vi "JSON Test.vi"() -> ()   [LabVIEW 2017]
uses:
  Classes/JSON Builder/JSON Builder.lvclass
  Typedefs/DSF Engine Framework Configuration.ctl
  DSF Core.lvlib
  Typedefs/DSF Engine Plugin Configuration.ctl
  Typedefs/DSF Timing Info.ctl
  Typedefs/DSF Engine Plugin Thread Configuration.ctl
  Typedefs/DSF Settings Info.ctl
  Typedefs/DSF Engine Transfer Group Configuration.ctl
  Typedefs/DSF Direction.ctl
  Typedefs/DSF Engine Transfer Configuration.ctl
  Typedefs/DSF Byte Order.ctl
  Typedefs/DSF Engine Channel Configuration.ctl
  Typedefs/DSF Data Type.ctl
  Typedefs/DSF Timeout Behavior.ctl
panel:
  out "Framework Configuration out":T1
  in  "Framework Configuration in":T1={"Plugins"=[{"name"="UDP", "components"=["UDP"], "cycle timing"={"priority"=100, "decimation"=1, "offset"=0}, "threads"=[{"buffer converter settings"=[], "transceiver settings"=[{"key"="Local Port", "value"="50000"}], "custom settings"=[], "processor"=-2, "priority offset"=0}, {"buffer converter settings"=[], "transceiver settings"=[{"key"="Local Port", "value"="50001"}], "custom settings"=[], "processor"=-2, "priority offset"=0}, {"buffer converter settings"=[], "transceiver settings"=[{"key"="Local Port", "value"="50002"}], "custom settings"=[], "processor"=-2, "priority offset"=0}, {"buffer converter settings"=[], "transceiver settings"=[{"key"="Local Port", "value"="50003"}], "custom settings"=[], "processor"=-2, "priority offset"=0}], "Transfer Groups"=[{"name"="Group", "direction"=enum."Tx", "cycle timing"={"priority"=100, "decimation"=1, "offset"=0}, "thread index"=0, "settings"=[], "Transfers"=[{"name"="Transfer", "byte order"=enum."big-endian", "settings"=[{"key"="Destination Port", "value"="60000"}, {"key"="Destination Address", "value"="localhost"}], "channels"=array[1000000 elements]}], "timeout behavior"=enum."Increment Late Count"}], "settings"=[]}]}
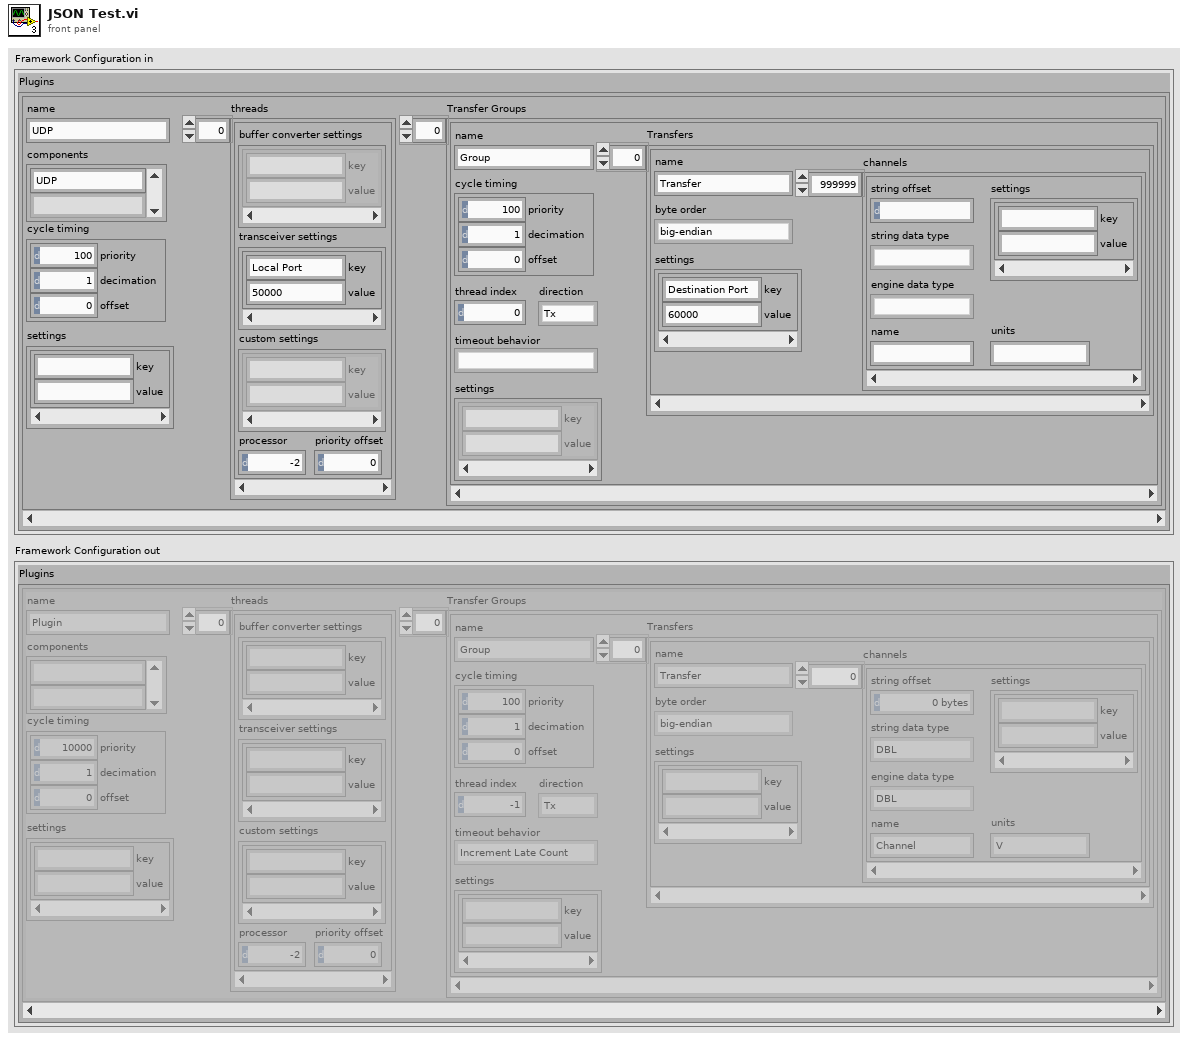
[diagram p1: front panel]
types:
  T1 = typedef "DSF Core.lvlib/DSF Engine Framework Configuration.ctl" = cluster{"Plugins":T2[]}
  T2 = typedef "DSF Core.lvlib/DSF Engine Plugin Configuration.ctl" = cluster{"name":string, "components":string[], "cycle timing":T3, "threads":T4[], "Transfer Groups":T6[], "settings":T5}
  T3 = typedef "DSF Core.lvlib/DSF Timing Info.ctl" = cluster{"priority":u64, "decimation":u64, "offset":u64}
  T4 = typedef "DSF Core.lvlib/DSF Engine Plugin Thread Configuration.ctl" = cluster{"buffer converter settings":T5, "transceiver settings":T5, "custom settings":T5, "processor":i32, "priority offset":i16}
  T5 = typedef "DSF Core.lvlib/DSF Settings Info.ctl" = cluster{"key":string, "value":string}[]
  T6 = typedef "DSF Core.lvlib/DSF Engine Transfer Group Configuration.ctl" = cluster{"name":string, "direction":T7, "cycle timing":T3, "thread index":i32, "settings":T5, "Transfers":T8[], "timeout behavior":T12}
  T7 = typedef "DSF Core.lvlib/DSF Direction.ctl" = enum8{"Tx", "Rx"}
  T8 = typedef "DSF Core.lvlib/DSF Engine Transfer Configuration.ctl" = cluster{"name":string, "byte order":T9, "settings":T5, "channels":T10[]}
  T9 = typedef "DSF Core.lvlib/DSF Byte Order.ctl" = enum8{"big-endian", "little-endian"}
  T10 = typedef "DSF Core.lvlib/DSF Engine Channel Configuration.ctl" = cluster{"string offset":u64, "string data type":T11, "engine data type":T11, "name":string, "settings":T5, "units":string}
  T11 = typedef "DSF Core.lvlib/DSF Data Type.ctl" = enum8{"Bool", "SGL", "DBL", "I8", "I16", "I32", "I64", "U8", "U16", "U32", "U64"}
  T12 = typedef "DSF Core.lvlib/DSF Timeout Behavior.ctl" = enum8{"Increment Late Count", "Throw Error"}
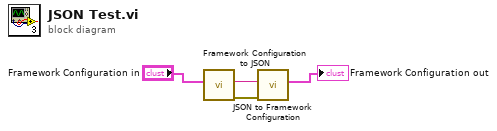
[diagram p0: block diagram]
diagram:
  n1 = call-dynamic "Framework Configuration to JSON.vi"("framework configuration"="Framework Configuration in") -> ("error out"=w3:errorcluster, "JSON string"=w4:string)  [unwired: 8 in, 1 out]
  n2 = call-dynamic "JSON to Framework Configuration.vi"("error in (no error)"=w3, "JSON string"=w4) -> ("Framework Configuration"=→"Framework Configuration out":T1)  [unwired: 7 in, 2 out]
